vi "Begin.vi"(8 "error in":errorcluster) -> (0 "error out":errorcluster)   [LabVIEW 2015]
doc: "Called before other user functions, this VI is expected to open initial I/O refnums, load in file data, and do all program initialization. Notice that the <B>error out</B> terminal is simply used for data flow. Wiring it to other structures or subVIs ensures that this VI runs first."
uses:
  <vilib>/Rock Robotics/WPI/DriverStation/WPI_DriverStationRobotMode2.ctl
  <vilib>/Rock Robotics/WPI/Joystick/WPI_JoystickDeviceEnum.ctl
  <vilib>/Rock Robotics/WPI/Solenoid/WPI_SolenoidChannel.ctl
  <vilib>/Rock Robotics/SystemInterfaces/AI/FPGA_AIChannel.ctl
  <vilib>/Rock Robotics/SystemInterfaces/DIO/FPGA_DIOChannel.ctl
  <vilib>/Rock Robotics/WPI/CAN/TalonSRX/WPI_CANTalonSRX_APIControlMode.ctl
  <vilib>/Rock Robotics/WPI/CAN/TalonSRX/WPI_CANTalonSRX_BrakeOverride.ctl
  <vilib>/Rock Robotics/SystemInterfaces/i2clib/i2c_bus.ctl
  <vilib>/Rock Robotics/WPI/AnalogOutput/WPI_AnalogOutputChannel.ctl
  navX-MXP Library/COMMON/TypeDefs/Value TypeDefs/navX Update Rate.ctl
  navX-MXP Library/COMMON/TypeDefs/Value TypeDefs/navX Interface Protocol.ctl
  <vilib>/Rock Robotics/SystemInterfaces/spilib/spi_bus.ctl
  Robot Global Data.vi
  <vilib>/Rock Robotics/WPI/Solenoid/WPI_SolenoidOpenSingle.vi
  <vilib>/Rock Robotics/WPI/Counter/WPI_CounterDigitalInputToDigitalSource.vi
  <vilib>/Rock Robotics/WPI/MotorControl/WPI_MotorControlOpenCANTalonSRX.vi
  <vilib>/Rock Robotics/WPI/Ultrasonic/WPI_SonarSRF04DigitalOpen.vi
  <vilib>/Rock Robotics/WPI/Ultrasonic/WPI_SonarSRF04DigitalRefNum Registry Set.vi
  <vilib>/Rock Robotics/WPI/Utilities/WPI_GetSetVariantRefNum.vi
  <vilib>/Rock Robotics/WPI/Camera/WPI_CameraWhite Balance Values.ctl
  <vilib>/Rock Robotics/WPI/Camera/WPI_CameraExposure Values.ctl
  <vilib>/Rock Robotics/WPI/Accelerometer/ADXL345 Range.ctl
  <vilib>/Rock Robotics/WPI/Accelerometer/WPI_AccelerometerADXL345 Axes.ctl
  <vilib>/Rock Robotics/WPI/RobotDrive/WPI_RobotDriveOpen2MotorWithExistingMotors.vi
  navX-MXP Library/navX-MXP IMU.lvlib
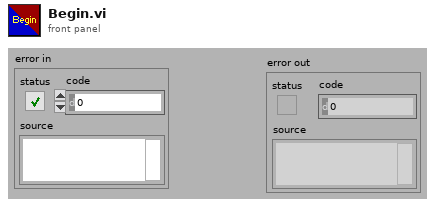
[diagram p1: front panel]
types:
  T1 = typedef "FPGA_AIChannel.ctl" = enum8{"AI 0", "AI 1", "AI 2", "AI 3", "AI MXP 0", "AI MXP 1", "AI MXP 2", "AI MXP 3", "Invalid"}
  T2 = typedef "FPGA_DIOChannel.ctl" = enum8{"DIO 0", "DIO 1", "DIO 2", "DIO 3", "DIO 4", "DIO 5", "DIO 6", "DIO 7", "DIO 8", "DIO 9", "DIO MXP 0", "DIO MXP 1", "DIO MXP 2", "DIO MXP 3", "DIO MXP 4", "DIO MXP 5", "DIO MXP 6", "DIO MXP 7", "DIO MXP 8", "DIO MXP 9", "DIO MXP 10", "DIO MXP 11", "DIO MXP 12", "DIO MXP 13", "DIO MXP 14", "DIO MXP 15", "Invalid"}
  T3 = typedef "WPI_AnalogOutputChannel.ctl" = enum8{"AO MXP 0", "AO MXP 1", "Invalid"}
  T4 = typedef "i2c_bus.ctl" = enum16{"I2C On-Board", "I2C MXP", "Invalid"}
  T5 = typedef "WPI_SolenoidChannel.ctl" = enum8{"Solenoid 0", "Solenoid 1", "Solenoid 2", "Solenoid 3", "Solenoid 4", "Solenoid 5", "Solenoid 6", "Solenoid 7", "Invalid"}
  T6 = typedef "WPI_CANTalonSRX_BrakeOverride.ctl" = enum8{"No Override", "Override to Coast", "Override to Brake"}
  T7 = typedef "WPI_CANTalonSRX_APIControlMode.ctl" = enum8{"Percent VBus", "Speed", "Position", "Slave", "Unchanged / Invalid", "Voltage Compensation", "Current", "Motion Profile"}
  T8 = typedef "WPI_JoystickDeviceEnum.ctl" = enum16{"USB 0", "USB 1", "USB 2", "USB 3", "USB 4", "USB 5"}
  T9 = typedef "WPI_DriverStationRobotMode2.ctl" = enum16{"Autonomous Disabled", "Autonomous Enabled", "Teleop Disabled", "Teleop Enabled", "Disconnected", "Finish", "Test Disabled", "Test Enabled", "Emergency Stopped"}
  T10 = typedef "WPI_CameraExposure Values.ctl" = enum16{"Auto", "Flicker-free 50 Hz", "Flicker-free 60 Hz", "Hold current", "Custom"}
  T11 = typedef "WPI_CameraWhite Balance Values.ctl" = enum16{"Auto", "Fixed indoor", "Fixed outdoor 1", "Fixed outdoor 2", "Fixed fluorescent 1", "Fixed fluorescent 2", "Hold current", "Custom"}
  T12 = typedef "WPI_CameraDevRef.ctl" = cluster{"Camera Address":string, "CameraStatus":errorcluster}
  T13 = typedef "WPI_SolenoidDevRef.ctl" = cluster{"DevStatus":errorcluster, "Pneumatics Control Module":u8, "Forward Solenoid Channel":T5, "Reverse Solenoid Channel":T5}
  T14 = typedef "WPI_MotorControlDeviceRef.ctl" = cluster{"DeviceStatus":errorcluster, "Type":T15, "PWM":cluster{"PWM Channel":T16, "DeadBand":T17}, "CAN":cluster{"Device Number":u8, "Control Mode":T18, "Semaphore":T19, "Max Vout":dbl, "TalonSRX Control Mode":T7}, "Invert":bool}
  T15 = typedef "WPI_MotorControlType.ctl" = enum16{"PWM", "CAN", "CANTalonSRX"}
  T16 = typedef "FPGA_DIOPWMChannel.ctl" = enum8{"PWM 0", "PWM 1", "PWM 2", "PWM 3", "PWM 4", "PWM 5", "PWM 6", "PWM 7", "PWM 8", "PWM 9", "PWM MXP 0", "PWM MXP 1", "PWM MXP 2", "PWM MXP 3", "PWM MXP 4", "PWM MXP 5", "PWM MXP 6", "PWM MXP 7", "PWM MXP 8", "PWM MXP 9", "Invalid"}
  T17 = typedef "WPI_PWMDeadband.ctl" = cluster{"Name":string, "maxPositivePwm":i32, "minPositivePwm":i32, "centerPwm":i32, "maxNegativePwm":i32, "minNegativePwm":i32, "angularRange":u16}
  T18 = typedef "WPI_CANJaguar_ControlMode.ctl" = enum8{"Percent VBus", "Current", "Speed", "Position", "Voltage"}
  T19 = typedef "Semaphore RefNum" = refnum<k1>
  T20 = typedef "WPI_DigitalInputDevRef.ctl" = cluster{"DevStatus":errorcluster, "DIO Channel":T2}
  T21 = typedef "WPI_CompressorDevRef.ctl" = cluster{"DevStatus":errorcluster, "Pneumatics Control Module":u8}
  T22 = typedef "FPGA_CounterEncoderSourceConvertionLVSourceType.ctl" = cluster{"DevStatus":errorcluster, "AnalogTriggerMode?":bool, "DigitalMode":cluster{"DIO Channel":T23}, "AnalogTriggerMode":cluster{"AnalogTriggerIndex":T24, "OutputType":T25}}
  T23 = typedef "FPGA_DIODigitalSourceChannel.ctl" = enum8{"DIO 0", "DIO 1", "DIO 2", "DIO 3", "DIO 4", "DIO 5", "DIO 6", "DIO 7", "DIO 8", "DIO 9", "DIO MXP 0", "DIO MXP 1", "DIO MXP 2", "DIO MXP 3", "DIO MXP 4", "DIO MXP 5", "DIO MXP 6", "DIO MXP 7", "DIO MXP 8", "DIO MXP 9", "DIO MXP 10", "DIO MXP 11", "DIO MXP 12", "DIO MXP 13", "DIO MXP 14", "DIO MXP 15", "Disabled"}
  T24 = typedef "FPGA_AnalogTriggerIndex.ctl" = enum8{"Trig 0", "Trig 1", "Trig 2", "Trig 3", "Trig 4", "Trig 5", "Trig 6", "Trig 7", "Invalid"}
  T25 = typedef "FPGA_AnalogTriggerOutType.ctl" = enum16{"InWindow", "TriggerState", "Rising", "Falling"}
  T26 = typedef "WPI_EncoderDevRef.ctl" = cluster{"DevStatus":errorcluster, "EncoderIndex":T27, "CounterIndex":T28, "DistancePerCount":dbl, "Decoding Type":T29}
  T27 = typedef "FPGA_EncoderIdx.ctl" = enum8{"Enc 0", "Enc 1", "Enc 2", "Enc 3", "Enc 4", "Enc 5", "Enc 6", "Enc 7", "Invalid"}
  T28 = typedef "FPGA_CounterCtrSystemIndex.ctl" = enum8{"Ctr 0", "Ctr 1", "Ctr 2", "Ctr 3", "Ctr 4", "Ctr 5", "Ctr 6", "Ctr 7", "Invalid"}
  T29 = typedef "WPI_EncoderType.ctl" = enum16{"1x", "2x", "4x"}
  T30 = typedef "WPI_AccelerometerADXL345 Axes.ctl" = cluster{"X-Axis":bool, "Y-Axis":bool, "Z-Axis":bool}
  T31 = typedef "spi_bus.ctl" = enum16{"SPI On-Board, CS0", "SPI On-Board, CS1", "SPI On-Board, CS2", "SPI On-Board, CS3", "SPI MXP", "Invalid"}
  T32 = typedef "navX-MXP IMU.lvlib/navX Interface Protocol.ctl" = enum16{"SPI", "I2C"}
  T33 = typedef "navX-MXP IMU.lvlib/navX Update Rate.ctl" = u8
  T34 = typedef "WPI_I2CDevRef.ctl" = cluster{"DevStatus":errorcluster, "Device Address":u8, "Handle":i32, "I2C Bus":T4}
  T35 = typedef "ADXL345 Range.ctl" = u8
  T36 = typedef "WPI_AccelerometerDevRef.ctl" = cluster{"DevStatus":errorcluster, "Scaling":T37, "Analog Channels":T38, "I2C Bus":T4, "SPI Bus":T31, "Accel Range":T35, "ADXL Axes":T30, "Handle":i32, "Device Address":u8, "Accel Type":enum16{"Analog", "ADXL345 I2C", "ADXL345 SPI", "Internal", "ADXL362 SPI"}}
  T37 = typedef "WPI_AccelerometerScaling.ctl" = cluster{"Gain (VoltsPerG)":dbl, "Center Voltage":dbl}
  T38 = typedef "WPI_AccelerometerAnalogChannels.ctl" = cluster{"X-Axis":T1, "Y-Axis":T1, "Z-Axis":T1}
  T39 = typedef "navX-MXP IMU.lvlib/navX Device TypeDef.ctl" = cluster{"navX Interface Protocol":T32, "navX Interface Protocol TypeDefs":cluster{"SPIDevRef":T40, "I2CDevRef":T34}, "navX System Information":cluster{"Board Information":T41, "Status":T42, "Offsets":T46}, "navX Common Information":cluster{"Update Rate (4Hz-60Hz)":T33, "refnum name":string, "error":errorcluster}}
  T40 = typedef "WPI_SPIDevRef.ctl" = cluster{"DevStatus":errorcluster, "Handle":i32, "SPI Bus":T31}
  T41 = typedef "navX-MXP IMU.lvlib/navX Board Information.ctl" = cluster{"WhoAmI (50 | 0x32)":u8, "Board Revision":u8, "Firmware Major Version":u8, "Firmware Minor Version":u8}
  T42 = typedef "navX-MXP IMU.lvlib/navX Status Data.ctl" = cluster{"Update Rate Hz":u8, "Accelerometer Full-Scale Range":u8, "Gyro Full-Scale Range":u16, "NAVX_OP_STATUS":T43, "NAVX_CAL_STATUS":T44, "NAVX_SELFTEST_STATUS":u8, "NAVX_SENSOR_STATUS":T45}
  T43 = typedef "navX-MXP IMU.lvlib/navX NAVX_OP_STATUS.ctl" = u8
  T44 = typedef "navX-MXP IMU.lvlib/navX NAVX_CAL_STATUS.ctl" = u8
  T45 = typedef "navX-MXP IMU.lvlib/navX NAVX_SENSOR_STATUS.ctl" = cluster{"MOVING":bool, "YAW_STABLE":bool, "MAG_DISTURBANCE":bool, "ALTITUDE_VALID":bool, "SEALEVEL_PRESS_SET":bool, "FUSED_HEADING_VALID":bool}
  T46 = typedef "navX-MXP IMU.lvlib/navX Offsets Data.ctl" = cluster{"Yaw":dbl, "Quat W":dbl, "Quat X":dbl, "Quat Y":dbl, "Quat Z":dbl}
  T47 = typedef "WPI_AnalogChannelDevRef.ctl" = cluster{"DevStatus":errorcluster, "Analog Channel":T1}
  T48 = typedef "WPI_PotentiometerDevRef.ctl" = cluster{"DevStatus":errorcluster, "Analog Channel":T1, "Invert Output":bool}
  T49 = typedef "WPI_JoystickDevRef.ctl" = cluster{"Device":T8}
  T50 = typedef "WPI_RobotDriveDevRef.ctl" = cluster{"DevStatus":errorcluster, "Motors[]":T14[], "Square Inputs":bool, "Max Output":dbl}
  T51 = typedef "WPI_UltrasonicDeviceRef.ctl" = cluster{"DevStatus":errorcluster, "Ping Channel":T2, "Echo Channel":T2, "CntIndex":T28}
  T52 = typedef "WPI_AOChannelDevRef.ctl" = cluster{"DevStatus":errorcluster, "AO Channel":T3}
  T53 = typedef "WPI_DigitalOutputDevRef.ctl" = cluster{"DIO Channel":T2, "DevStatus":errorcluster}
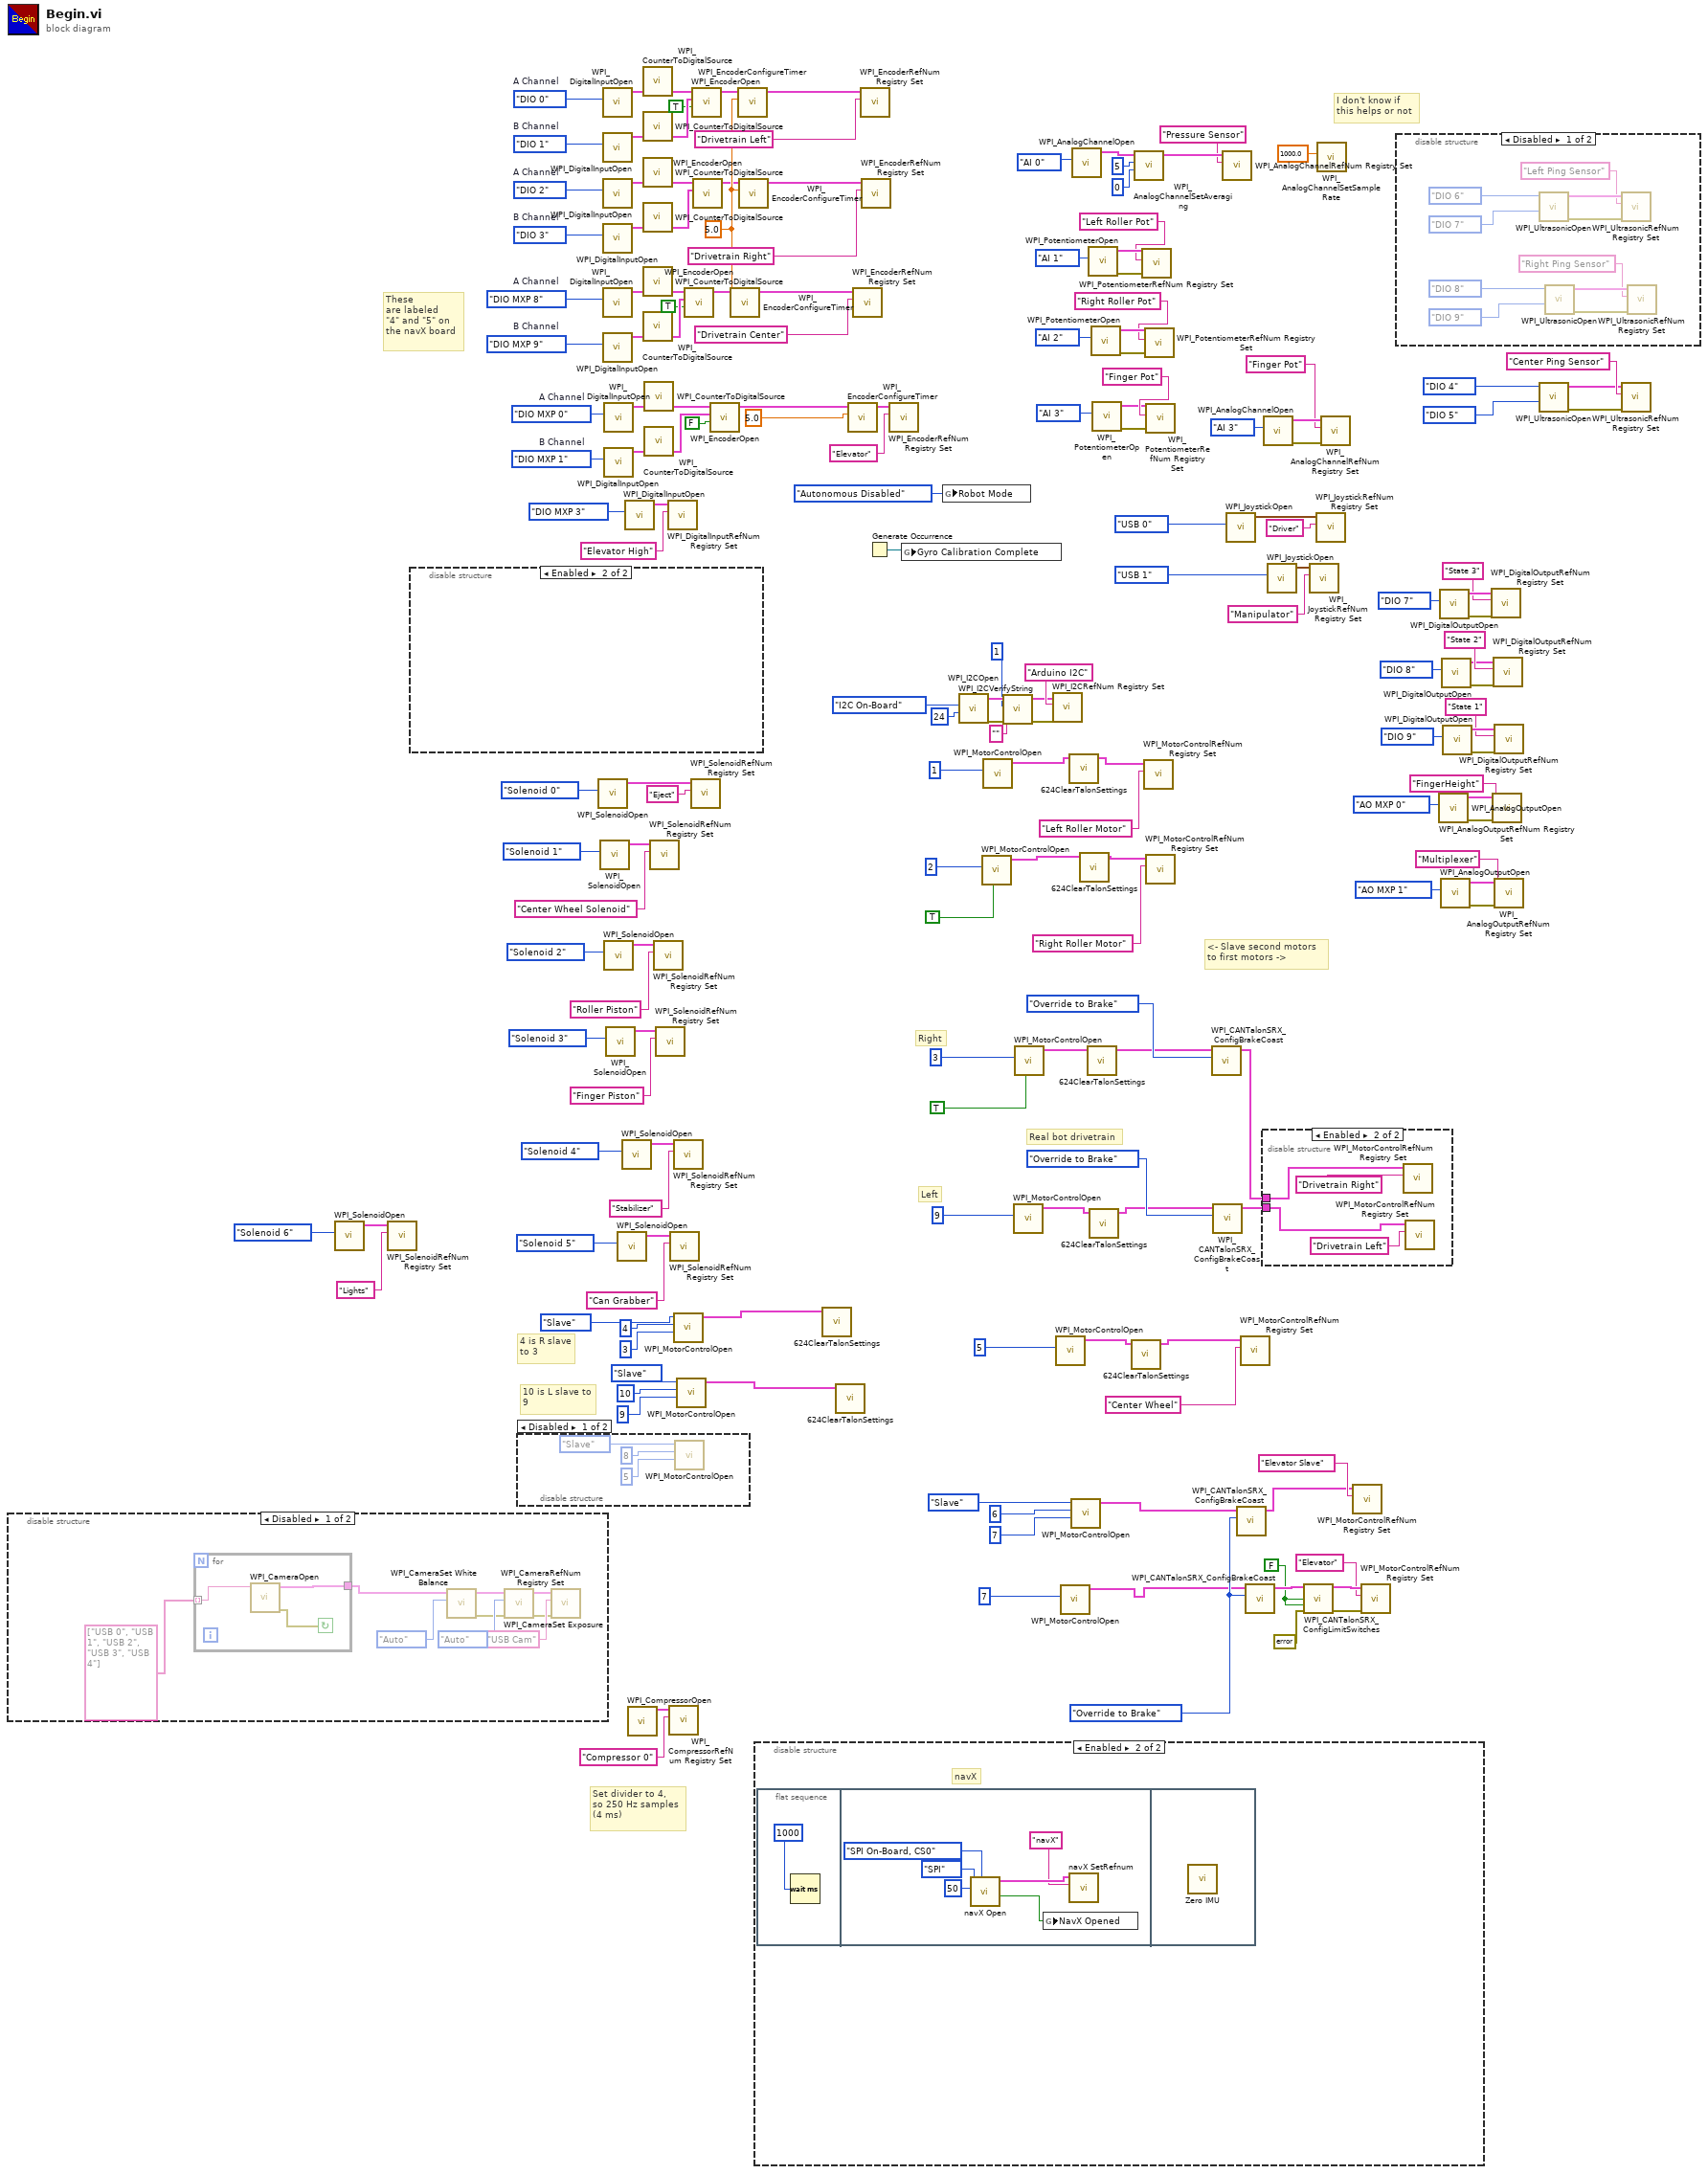
[diagram p0: block diagram]
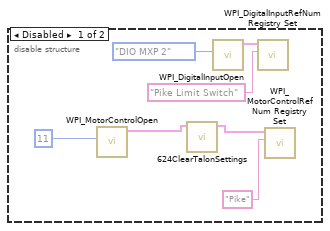
[diagram p2: hidden frame]
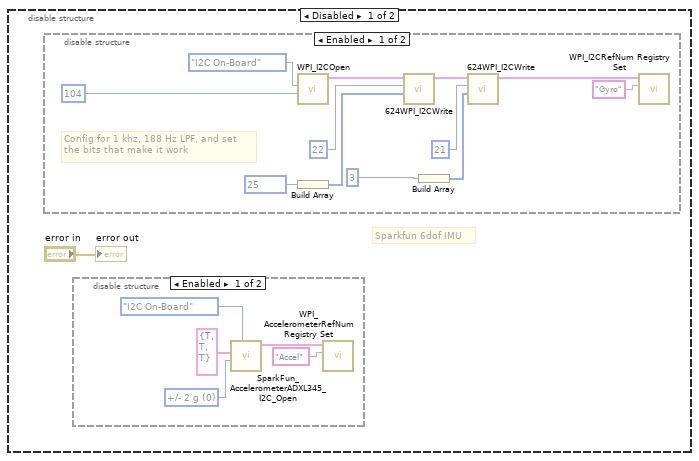
[diagram p5: hidden frame]
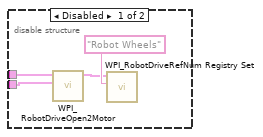
[diagram p9: hidden frame]
diagram:
  w41 = FPGA_DIOChannel."DIO MXP 9"  # B Channel
  w42 = FPGA_DIOChannel."DIO MXP 8"  # A Channel
  w66 = FALSE ("Forward Limit Switch Normally Open")
  w64 = WPI_CANTalonSRX_BrakeOverride."Override to Brake" ("Brake / Coast Mode")
  w94 = FPGA_DIOChannel."DIO MXP 1"  # B Channel
  w95 = FPGA_DIOChannel."DIO MXP 0"  # A Channel
  w122 = FPGA_DIOChannel."DIO 3"  # B Channel
  w125 = FPGA_DIOChannel."DIO 2"  # A Channel
  w131 = FPGA_DIOChannel."DIO 0"  # A Channel
  w134 = FPGA_DIOChannel."DIO 1"  # B Channel
  w139 = 5.0 ("Minimum Rate")
  # "10 is L slave to\n9"
  # "4 is R slave\nto 3"
  # "These \nare labeled\n\"4\" and \"5\" on \nthe navX board"
  # "<- Slave second motors\nto first motors ->"
  # "Left"
  # "Right"
  # "Real bot drivetrain"
  # "I don't know if \nthis helps or not"
  # "Set divider to 4, \nso 250 Hz samples\n(4 ms)"
  n1 = disable-structure shown="Disabled" {
    frame Disabled {
      n2 = for {
        tunnel: string[] ["USB 0", "USB 1", "USB 2", "USB 3", "USB 4"] -> [w191] mode=indexing
        tunnel: [w190] -> w180
        stop <- w189 continue-if-true
        n3 = call <vilib>:"WPI_CameraOpen.vi"("Camera Address"=w191) -> ("error out"=w189:errorcluster, "CameraDevRef"=w190:T12)  [unwired: 9 in]
      }
      n4 = call <vilib>:"WPI_CameraSet White Balance.vi"("White Balance"=WPI_CameraWhite_Balance_Values."Auto", "CameraDevRef"=w180) -> ("error out"=w183:errorcluster, "CameraDevRef Out"=w187:T12)  [unwired: 8 in]
      n5 = call <vilib>:"WPI_CameraSet Exposure.vi"("error in (no error)"=w183, "Exposure"=WPI_CameraExposure_Values."Auto", "CameraDevRef"=w187) -> ("error out"=w182:errorcluster, "CameraDevRef Out"=w185:T12)  [unwired: 7 in]
      n6 = call <vilib>:"WPI_CameraRefNum Registry Set.vi"("error in (no error)"=w182, "refnum name"="USB Cam", "CameraDevRef"=w185) -> ()  [unwired: 7 in, 2 out]
    }
    frame Enabled {
    }
  }
  n7 = call-poly <vilib>:"WPI_SolenoidOpen.vi"("Solenoid Channel"=WPI_SolenoidChannel."Solenoid 6") -> ("SolenoidDevRef"=w39:T13)  [unwired: 9 in, 1 out]
  n8 = call <vilib>:"WPI_SolenoidRefNum Registry Set.vi"("refnum name"="Lights", "SolenoidDevRef"=w39) -> ()  [unwired: 8 in, 2 out]
  n9 = disable-structure shown="Enabled" {
    frame Disabled {
      n10 = call-poly <vilib>:"WPI_MotorControlOpen.vi"("Device Number"=u8 11) -> ("MotorControlDeviceRef"=w194:T14)  [unwired: 9 in, 1 out]
      n11 = call "624ClearTalonSettings.vi"("CAN Talon SRX Ref Out"=w194) -> ("CAN Talon SRX Ref Out 2"=w193:T14)  [unwired: 10 in]
      n12 = call <vilib>:"WPI_DigitalInputOpen.vi"("DIO Channel"=FPGA_DIOChannel."DIO MXP 2") -> ("DigitalInputDevRef"=w196:T20)  [unwired: 9 in, 1 out]
      n13 = call <vilib>:"WPI_DigitalInputRefNum Registry Set.vi"("refnum name"="Pike Limit Switch", "DigitalInputDevRef"=w196) -> ()  [unwired: 8 in, 2 out]
      n14 = call <vilib>:"WPI_MotorControlRefNum Registry Set.vi"("refnum name"="Pike", "MotorControlDevRef"=w193) -> ()  [unwired: 8 in, 2 out]
    }
    frame Enabled {
    }
  }
  n15 = disable-structure shown="Disabled" {
    frame Disabled {
      n16 = call-poly <vilib>:"WPI_MotorControlOpen.vi"("Master Device Number"=u8 5, "Device Number"=u8 8, "Control Mode"=WPI_CANTalonSRX_APIControlMode."Slave") -> ()  [unwired: 7 in, 2 out]
    }
    frame Enabled {
    }
  }
  n17 = call-poly <vilib>:"WPI_SolenoidOpen.vi"("Solenoid Channel"=WPI_SolenoidChannel."Solenoid 0") -> ("SolenoidDevRef"=w108:T13)  [unwired: 9 in, 1 out]
  n18 = call-poly <vilib>:"WPI_SolenoidOpen.vi"("Solenoid Channel"=WPI_SolenoidChannel."Solenoid 1") -> ("SolenoidDevRef"=w107:T13)  [unwired: 9 in, 1 out]
  n19 = call <vilib>:"WPI_DigitalInputOpen.vi"("DIO Channel"=w131) -> ("DigitalInputDevRef"=w132:T20)  [unwired: 1 in, 9 out]
  n20 = call <vilib>:"WPI_DigitalInputOpen.vi"("DIO Channel"=w134) -> ("DigitalInputDevRef"=w135:T20)  [unwired: 1 in, 9 out]
  n21 = call <vilib>:"WPI_DigitalInputOpen.vi"("DIO Channel"=w125) -> ("DigitalInputDevRef"=w126:T20)  [unwired: 1 in, 9 out]
  n22 = call <vilib>:"WPI_DigitalInputOpen.vi"("DIO Channel"=w122) -> ("DigitalInputDevRef"=w123:T20)  [unwired: 1 in, 9 out]
  n23 = call <vilib>:"WPI_DigitalInputOpen.vi"("DIO Channel"=w42) -> ("DigitalInputDevRef"=w140:T20)  [unwired: 1 in, 9 out]
  n24 = call <vilib>:"WPI_DigitalInputOpen.vi"("DIO Channel"=w41) -> ("DigitalInputDevRef"=w142:T20)  [unwired: 1 in, 9 out]
  n25 = call <vilib>:"WPI_DigitalInputOpen.vi"("DIO Channel"=w95) -> ("DigitalInputDevRef"=w156:T20)  [unwired: 1 in, 9 out]
  n26 = call <vilib>:"WPI_DigitalInputOpen.vi"("DIO Channel"=w94) -> ("DigitalInputDevRef"=w158:T20)  [unwired: 1 in, 9 out]
  n27 = call-poly <vilib>:"WPI_SolenoidOpen.vi"("Solenoid Channel"=WPI_SolenoidChannel."Solenoid 2") -> ("SolenoidDevRef"=w109:T13)  [unwired: 9 in, 1 out]
  n28 = call-poly <vilib>:"WPI_SolenoidOpen.vi"("Solenoid Channel"=WPI_SolenoidChannel."Solenoid 3") -> ("SolenoidDevRef"=w111:T13)  [unwired: 9 in, 1 out]
  n29 = call-poly <vilib>:"WPI_SolenoidOpen.vi"("Solenoid Channel"=WPI_SolenoidChannel."Solenoid 5") -> ("SolenoidDevRef"=w45:T13)  [unwired: 9 in, 1 out]
  n30 = call-poly <vilib>:"WPI_SolenoidOpen.vi"("Solenoid Channel"=WPI_SolenoidChannel."Solenoid 4") -> ("SolenoidDevRef"=w114:T13)  [unwired: 9 in, 1 out]
  n31 = call <vilib>:"WPI_DigitalInputOpen.vi"("DIO Channel"=FPGA_DIOChannel."DIO MXP 3") -> ("DigitalInputDevRef"=w164:T20)  [unwired: 9 in, 1 out]
  n32 = call <vilib>:"WPI_CompressorOpen.vi"() -> ("CompressorDevRef"=w173:T21)  [unwired: 14 in, 1 out]
  n33 = call-poly <vilib>:"WPI_CounterToDigitalSource.vi"("DigitalInputDevRef"=w132) -> ("Digital Source"=w133:T22)  [unwired: 6 out]
  n34 = call-poly <vilib>:"WPI_CounterToDigitalSource.vi"("DigitalInputDevRef"=w135) -> ("Digital Source"=w136:T22)  [unwired: 6 out]
  n35 = call-poly <vilib>:"WPI_CounterToDigitalSource.vi"("DigitalInputDevRef"=w126) -> ("Digital Source"=w127:T22)  [unwired: 6 out]
  n36 = call-poly <vilib>:"WPI_CounterToDigitalSource.vi"("DigitalInputDevRef"=w123) -> ("Digital Source"=w124:T22)  [unwired: 6 out]
  n37 = call-poly <vilib>:"WPI_CounterToDigitalSource.vi"("DigitalInputDevRef"=w140) -> ("Digital Source"=w141:T22)  [unwired: 6 out]
  n38 = call-poly <vilib>:"WPI_CounterToDigitalSource.vi"("DigitalInputDevRef"=w142) -> ("Digital Source"=w143:T22)  [unwired: 6 out]
  n39 = call-poly <vilib>:"WPI_CounterToDigitalSource.vi"("DigitalInputDevRef"=w156) -> ("Digital Source"=w157:T22)  [unwired: 6 out]
  n40 = call-poly <vilib>:"WPI_CounterToDigitalSource.vi"("DigitalInputDevRef"=w158) -> ("Digital Source"=w159:T22)  [unwired: 6 out]
  n41 = call <vilib>:"WPI_SolenoidRefNum Registry Set.vi"("refnum name"="Center Wheel Solenoid", "SolenoidDevRef"=w107) -> ()  [unwired: 8 in, 2 out]
  n42 = call <vilib>:"WPI_SolenoidRefNum Registry Set.vi"("refnum name"="Roller Piston", "SolenoidDevRef"=w109) -> ()  [unwired: 8 in, 2 out]
  n43 = call <vilib>:"WPI_SolenoidRefNum Registry Set.vi"("refnum name"="Finger Piston", "SolenoidDevRef"=w111) -> ()  [unwired: 8 in, 2 out]
  n44 = call <vilib>:"WPI_DigitalInputRefNum Registry Set.vi"("refnum name"="Elevator High", "DigitalInputDevRef"=w164) -> ()  [unwired: 8 in, 2 out]
  n45 = call <vilib>:"WPI_CompressorRefNum Registry Set.vi"("refnum name"="Compressor 0", "CompressorDevRef"=w173) -> ()  [unwired: 8 in, 2 out]
  n46 = call <vilib>:"WPI_SolenoidRefNum Registry Set.vi"("refnum name"="Can Grabber", "SolenoidDevRef"=w45) -> ()  [unwired: 8 in, 2 out]
  n47 = call <vilib>:"WPI_SolenoidRefNum Registry Set.vi"("refnum name"="Stabilizer", "SolenoidDevRef"=w114) -> ()  [unwired: 8 in, 2 out]
  n48 = call-poly <vilib>:"WPI_MotorControlOpen.vi"("Master Device Number"=u8 3, "Device Number"=u8 4, "Control Mode"=WPI_CANTalonSRX_APIControlMode."Slave") -> ("MotorControlDeviceRef"=w53:T14)  [unwired: 7 in, 1 out]
  n49 = call-poly <vilib>:"WPI_MotorControlOpen.vi"("Master Device Number"=u8 9, "Device Number"=u8 10, "Control Mode"=WPI_CANTalonSRX_APIControlMode."Slave") -> ("MotorControlDeviceRef"=w52:T14)  [unwired: 7 in, 1 out]
  n50 = call <vilib>:"WPI_EncoderOpen.vi"("Invert Direction (False)"=TRUE, "BSource"=w143, "ASource"=w141) -> ("EncoderDevRef"=w144:T26)  [unwired: 5 in, 3 out]
  n51 = call <vilib>:"WPI_SolenoidRefNum Registry Set.vi"("refnum name"="Eject", "SolenoidDevRef"=w108) -> ()  [unwired: 8 in, 2 out]
  n52 = call <vilib>:"WPI_EncoderOpen.vi"("Invert Direction (False)"=TRUE, "BSource"=w136, "ASource"=w133) -> ("EncoderDevRef"=w137:T26)  [unwired: 5 in, 3 out]
  n53 = call <vilib>:"WPI_EncoderOpen.vi"("BSource"=w124, "ASource"=w127) -> ("EncoderDevRef"=w128:T26)  [unwired: 6 in, 3 out]
  n54 = call <vilib>:"WPI_EncoderOpen.vi"("Invert Direction (False)"=FALSE, "BSource"=w159, "ASource"=w157) -> ("EncoderDevRef"=w160:T26)  [unwired: 5 in, 3 out]
  n55 = call <vilib>:"WPI_EncoderConfigureTimer.vi"("Minimum Rate"=w139, "EncoderDevRef"=w144) -> ("EncoderDevRef"=w145:T26)  [unwired: 8 in, 1 out]
  n56 = call <vilib>:"WPI_EncoderConfigureTimer.vi"("Minimum Rate"=w139, "EncoderDevRef"=w137) -> ("EncoderDevRef"=w138:T26)  [unwired: 8 in, 1 out]
  n57 = call <vilib>:"WPI_EncoderConfigureTimer.vi"("Minimum Rate"=w139, "EncoderDevRef"=w128) -> ("EncoderDevRef"=w129:T26)  [unwired: 8 in, 1 out]
  n58 = disable-structure shown="Enabled" {
    frame Disabled {
      # "Sparkfun 6dof IMU"
      n59 = disable-structure shown="Enabled" {
        frame Enabled {
          # "Config for 1 khz, 188 Hz LPF, and set\nthe bits that make it work"
          n60 = call <vilib>:"WPI_I2COpen.vi"("Device Address"=104, "I2C Bus"=i2c_bus."I2C On-Board") -> ("I2CDevRef"=w218:T34)  [unwired: 8 in, 1 out]
          n61 = Build Array(u8 25) -> (w215:u8[])
          n62 = call "624WPI_I2CWrite.vi"("I2CDataToSend"=w215, "I2CRegister"=u8 22, "I2CDevRef"=w218) -> ("I2CDevRef"=w219:T34)  [unwired: 7 in, 1 out]
          n63 = Build Array(u8 3) -> (w212:u8[])
          n64 = call "624WPI_I2CWrite.vi"("I2CDataToSend"=w212, "I2CRegister"=u8 21, "I2CDevRef"=w219) -> ("I2CDevRef"=w208:T34)  [unwired: 7 in, 1 out]
          n65 = call <vilib>:"WPI_I2CRefNum Registry Set.vi"("refnum name"="Gyro", "I2CDevRef"=w208) -> ()  [unwired: 8 in, 2 out]
        }
        frame Disabled {
        }
      }
      n66 = disable-structure shown="Enabled" {
        frame Enabled {
          w206 = T35 0 items=["+/- 2 g", "+/- 4 g", "+/- 8 g", "+/- 16 g"] ("Accel Range")
          n67 = call "SparkFun_AccelerometerADXL345_I2C_Open.vi"("I2C Bus"=i2c_bus."I2C On-Board", "Accel Range"=w206, "ADXL345 Axes"=T30 {"X-Axis"=TRUE, "Y-Axis"=TRUE, "Z-Axis"=TRUE}) -> ("AccelerometerDevRef"=w207:T36)  [unwired: 7 in, 1 out]
          n68 = call <vilib>:"WPI_AccelerometerRefNum Registry Set.vi"("refnum name"="Accel", "AccelerometerDevRef"=w207) -> ()  [unwired: 8 in, 2 out]
        }
        frame Disabled {
        }
      }
      "error out" <- "error in"
    }
    frame Enabled {
      # "navX"
      n69 = flat-sequence {
        frame #0 {
          n70 = Wait (ms)(milliseconds to wait=u32 1000) -> ()  [unwired: 1 out]
        }
        frame #1 {
          n71 = call "navX Open.vi"("SPI Bus"=spi_bus."SPI On-Board, CS0", "Update Rate (4Hz-60Hz)"=T33 50, "navX Interface Protocol"=navX_Interface_Protocol."SPI") -> ("Opened?"=w224:bool, "navX Device TypeDef"=w226:T39)  [unwired: 6 in, 1 out]
          n72 = global write "Robot Global Data.vi" "NavX Opened"(w224) -> ()
          n73 = call "navX SetRefnum.vi"("refnum name"="navX", "navX Device TypeDef"=w226) -> ()  [unwired: 8 in, 2 out]
        }
        frame #2 {
          n74 = call "Zero IMU.vi"() -> ()  [unwired: 12 in]
        }
      }
    }
  }
  n75 = call "624ClearTalonSettings.vi"("CAN Talon SRX Ref Out"=w53) -> ()  [unwired: 10 in, 1 out]
  n76 = call "624ClearTalonSettings.vi"("CAN Talon SRX Ref Out"=w52) -> ()  [unwired: 10 in, 1 out]
  n77 = call <vilib>:"WPI_EncoderConfigureTimer.vi"("Minimum Rate"=5.0, "EncoderDevRef"=w160) -> ("EncoderDevRef"=w161:T26)  [unwired: 8 in, 1 out]
  n78 = call <vilib>:"WPI_EncoderRefNum Registry Set.vi"("refnum name"="Drivetrain Center", "EncoderDevRef"=w145) -> ()  [unwired: 8 in, 2 out]
  n79 = call <vilib>:"WPI_EncoderRefNum Registry Set.vi"("refnum name"="Drivetrain Left", "EncoderDevRef"=w138) -> ()  [unwired: 8 in, 2 out]
  n80 = call <vilib>:"WPI_EncoderRefNum Registry Set.vi"("refnum name"="Drivetrain Right", "EncoderDevRef"=w129) -> ()  [unwired: 8 in, 2 out]
  n81 = Generate Occurrence() -> (w48:refnum<k4>)
  n82 = call <vilib>:"WPI_EncoderRefNum Registry Set.vi"("refnum name"="Elevator", "EncoderDevRef"=w161) -> ()  [unwired: 8 in, 2 out]
  n83 = global write "Robot Global Data.vi" "Gyro Calibration Complete"(w48) -> ()
  n84 = global write "Robot Global Data.vi" "Robot Mode"(WPI_DriverStationRobotMode2."Autonomous Disabled" ("Robot Mode")) -> ()
  n85 = call <vilib>:"WPI_I2COpen.vi"("Device Address"=u8 24, "I2C Bus"=i2c_bus."I2C On-Board") -> ("error out"=w31:errorcluster, "I2CDevRef"=w34:T34)  [unwired: 8 in]
  n86 = call-poly <vilib>:"WPI_MotorControlOpen.vi"("Invert"=TRUE, "Device Number"=u8 2) -> ("MotorControlDeviceRef"=w56:T14)  [unwired: 8 in, 1 out]
  n87 = call-poly <vilib>:"WPI_MotorControlOpen.vi"("Device Number"=u8 1) -> ("MotorControlDeviceRef"=w54:T14)  [unwired: 9 in, 1 out]
  n88 = call <vilib>:"WPI_I2CVerifyString.vi"("error in (no error)"=w31, "Expected"="", "Register Address"=u8 1, "I2CDevRef"=w34) -> ("error out"=w32:errorcluster, "I2CDevRef"=w33:T34)  [unwired: 6 in]
  n89 = call-poly <vilib>:"WPI_MotorControlOpen.vi"("Device Number"=u8 9) -> ("MotorControlDeviceRef"=w60:T14)  [unwired: 9 in, 1 out]
  n90 = call-poly <vilib>:"WPI_MotorControlOpen.vi"("Invert"=TRUE, "Device Number"=u8 3) -> ("MotorControlDeviceRef"=w58:T14)  [unwired: 8 in, 1 out]
  n91 = call <vilib>:"WPI_I2CRefNum Registry Set.vi"("error in (no error)"=w32, "refnum name"="Arduino I2C", "I2CDevRef"=w33) -> ()  [unwired: 7 in, 2 out]
  n92 = call-poly <vilib>:"WPI_MotorControlOpen.vi"("Device Number"=u8 5) -> ("MotorControlDeviceRef"=w62:T14)  [unwired: 9 in, 1 out]
  n93 = call-poly <vilib>:"WPI_MotorControlOpen.vi"("Device Number"=u8 7) -> ("MotorControlDeviceRef"=w49:T14)  [unwired: 9 in, 1 out]
  n94 = call "624ClearTalonSettings.vi"("CAN Talon SRX Ref Out"=w54) -> ("CAN Talon SRX Ref Out 2"=w55:T14)  [unwired: 10 in]
  n95 = call-poly <vilib>:"WPI_MotorControlOpen.vi"("Master Device Number"=u8 7, "Device Number"=u8 6, "Control Mode"=WPI_CANTalonSRX_APIControlMode."Slave") -> ("MotorControlDeviceRef"=w50:T14)  [unwired: 7 in, 1 out]
  n96 = call <vilib>:"WPI_AnalogChannelOpen.vi"("Analog Channel"=FPGA_AIChannel."AI 0") -> ("AIDeviceRef"=w169:T47)  [unwired: 9 in, 1 out]
  n97 = call "624ClearTalonSettings.vi"("CAN Talon SRX Ref Out"=w56) -> ("CAN Talon SRX Ref Out 2"=w57:T14)  [unwired: 10 in]
  n98 = call "624ClearTalonSettings.vi"("CAN Talon SRX Ref Out"=w58) -> ("CAN Talon SRX Ref Out 2"=w59:T14)  [unwired: 10 in]
  n99 = call <vilib>:"WPI_PotentiometerOpen.vi"("Analog Channel"=FPGA_AIChannel."AI 1") -> ("error out"=w99:errorcluster, "PotDevRef"=w98:T48)  [unwired: 9 in]
  n100 = call "624ClearTalonSettings.vi"("CAN Talon SRX Ref Out"=w60) -> ("CAN Talon SRX Ref Out 2"=w61:T14)  [unwired: 10 in]
  n101 = call <vilib>:"WPI_PotentiometerOpen.vi"("Analog Channel"=FPGA_AIChannel."AI 2") -> ("error out"=w103:errorcluster, "PotDevRef"=w102:T48)  [unwired: 9 in]
  n102 = call <vilib>:"WPI_PotentiometerOpen.vi"("Analog Channel"=FPGA_AIChannel."AI 3") -> ("error out"=w1:errorcluster, "PotDevRef"=w2:T48)  [unwired: 9 in]
  n103 = call "624ClearTalonSettings.vi"("CAN Talon SRX Ref Out"=w62) -> ("CAN Talon SRX Ref Out 2"=w63:T14)  [unwired: 10 in]
  n104 = call <vilib>:"WPI_AnalogChannelSetAveraging.vi"("OversampleBits"=u8 0, "AverageBits"=u8 5, "AIDeviceRef"=w169) -> ("AIDeviceRef"=w170:T47)  [unwired: 7 in, 1 out]
  n105 = call <vilib>:"WPI_PotentiometerRefNum Registry Set.vi"("error in (no error)"=w99, "refnum name"="Left Roller Pot", "PotDevRef"=w98) -> ()  [unwired: 7 in, 2 out]
  n106 = call <vilib>:"WPI_MotorControlRefNum Registry Set.vi"("refnum name"="Left Roller Motor", "MotorControlDevRef"=w55) -> ()  [unwired: 8 in, 2 out]
  n107 = call <vilib>:"WPI_PotentiometerRefNum Registry Set.vi"("error in (no error)"=w103, "refnum name"="Right Roller Pot", "PotDevRef"=w102) -> ()  [unwired: 7 in, 2 out]
  n108 = call <vilib>:"WPI_PotentiometerRefNum Registry Set.vi"("error in (no error)"=w1, "refnum name"="Finger Pot", "PotDevRef"=w2) -> ()  [unwired: 7 in, 2 out]
  n109 = call <vilib>:"WPI_MotorControlRefNum Registry Set.vi"("refnum name"="Right Roller Motor", "MotorControlDevRef"=w57) -> ()  [unwired: 8 in, 2 out]
  n110 = call <vilib>:"WPI_CANTalonSRX_ConfigBrakeCoast.vi"("Brake / Coast Mode"=WPI_CANTalonSRX_BrakeOverride."Override to Brake", "CAN Talon SRX Ref"=w59) -> ("CAN Talon SRX Ref"=w82:T14)  [unwired: 8 in, 1 out]
  n111 = call <vilib>:"WPI_CANTalonSRX_ConfigBrakeCoast.vi"("Brake / Coast Mode"=WPI_CANTalonSRX_BrakeOverride."Override to Brake", "CAN Talon SRX Ref"=w61) -> ("CAN Talon SRX Ref"=w85:T14)  [unwired: 8 in, 1 out]
  n112 = call <vilib>:"WPI_AnalogChannelRefNum Registry Set.vi"("refnum name"="Pressure Sensor", "AIDeviceRef"=w170) -> ()  [unwired: 8 in, 2 out]
  n113 = call <vilib>:"WPI_JoystickOpen.vi"("JoystickDevice"=WPI_JoystickDeviceEnum."USB 0") -> ("JoystickDevRef"=w178:T49)  [unwired: 10 in]
  n114 = call <vilib>:"WPI_CANTalonSRX_ConfigBrakeCoast.vi"("Brake / Coast Mode"=w64, "CAN Talon SRX Ref"=w50) -> ("CAN Talon SRX Ref"=w46:T14)  [unwired: 8 in, 1 out]
  n115 = call <vilib>:"WPI_MotorControlRefNum Registry Set.vi"("refnum name"="Center Wheel", "MotorControlDevRef"=w63) -> ()  [unwired: 8 in, 2 out]
  n116 = call <vilib>:"WPI_CANTalonSRX_ConfigBrakeCoast.vi"("Brake / Coast Mode"=w64, "CAN Talon SRX Ref"=w49) -> ("CAN Talon SRX Ref"=w68:T14)  [unwired: 8 in, 1 out]
  n117 = disable-structure shown="Enabled" {
    disable-tunnel: w85 -> [w228 w231]
    disable-tunnel: w82 -> [w227 w234]
    frame Disabled {
      n118 = call-poly <vilib>:"WPI_RobotDriveOpen2Motor.vi"("Right Motor Dev Ref"=w228, "Left Motor Dev Ref"=w227) -> ("RobotDriveDevRef"=w229:T50)  [unwired: 8 in, 1 out]
      n119 = call <vilib>:"WPI_RobotDriveRefNum Registry Set.vi"("refnum name"="Robot Wheels", "RobotDriveDevRef"=w229) -> ()  [unwired: 8 in, 2 out]
    }
    frame Enabled {
      n120 = call <vilib>:"WPI_MotorControlRefNum Registry Set.vi"("refnum name"="Drivetrain Right", "MotorControlDevRef"=w234) -> ()  [unwired: 8 in, 2 out]
      n121 = call <vilib>:"WPI_MotorControlRefNum Registry Set.vi"("refnum name"="Drivetrain Left", "MotorControlDevRef"=w231) -> ()  [unwired: 8 in, 2 out]
    }
  }
  n122 = call <vilib>:"WPI_AnalogChannelOpen.vi"("Analog Channel"=FPGA_AIChannel."AI 3") -> ("error out"=w5:errorcluster, "AIDeviceRef"=w7:T47)  [unwired: 9 in]
  n123 = call <vilib>:"WPI_JoystickOpen.vi"("JoystickDevice"=WPI_JoystickDeviceEnum."USB 1") -> ("JoystickDevRef"=w151:T49)  [unwired: 10 in]
  n124 = call <vilib>:"WPI_CANTalonSRX_ConfigLimitSwitches.vi"("CAN Talon SRX Ref"=w68, "Forward Limit Switch Normally Open"=w66, "Reverse Limit Switch Normally Open"=w66, "error in (no error)"=errorcluster {"status"=FALSE, "code"=0, "source"=""}) -> ("CAN Talon SRX Ref"=w70:T14, "error out"=w69:errorcluster)  [unwired: 10 in]
  n125 = call <vilib>:"WPI_JoystickRefNum Registry Set.vi"("refnum name"="Manipulator", "JoystickDevRef"=w151) -> ()  [unwired: 8 in, 2 out]
  n126 = call <vilib>:"WPI_JoystickRefNum Registry Set.vi"("refnum name"="Driver", "JoystickDevRef"=w178) -> ()  [unwired: 8 in, 2 out]
  n127 = call <vilib>:"WPI_AnalogChannelSetSampleRate.vi"("Samples Per Second (per channel)"=1000.0) -> ()  [unwired: 10 in, 1 out]
  n128 = call <vilib>:"WPI_AnalogChannelRefNum Registry Set.vi"("error in (no error)"=w5, "refnum name"="Finger Pot", "AIDeviceRef"=w7) -> ()  [unwired: 7 in, 2 out]
  n129 = call <vilib>:"WPI_MotorControlRefNum Registry Set.vi"("refnum name"="Elevator Slave", "MotorControlDevRef"=w46) -> ()  [unwired: 8 in, 2 out]
  n130 = call <vilib>:"WPI_MotorControlRefNum Registry Set.vi"("error in (no error)"=w69, "refnum name"="Elevator", "MotorControlDevRef"=w70) -> ()  [unwired: 7 in, 2 out]
  n131 = disable-structure shown="Disabled" {
    frame Disabled {
      n132 = call-poly <vilib>:"WPI_UltrasonicOpen.vi"("Echo DIO Channel"=FPGA_DIOChannel."DIO 7", "Ping DIO Channel"=FPGA_DIOChannel."DIO 6") -> ("error out"=w239:errorcluster, "SonarSRF04DevRef"=w238:T51)  [unwired: 8 in]
      n133 = call-poly <vilib>:"WPI_UltrasonicOpen.vi"("Echo DIO Channel"=FPGA_DIOChannel."DIO 9", "Ping DIO Channel"=FPGA_DIOChannel."DIO 8") -> ("error out"=w244:errorcluster, "SonarSRF04DevRef"=w243:T51)  [unwired: 8 in]
      n134 = call-poly <vilib>:"WPI_UltrasonicRefNum Registry Set.vi"("error in (no error)"=w239, "refnum name"="Left Ping Sensor", "SonarSRF04DevRef"=w238) -> ()  [unwired: 7 in, 2 out]
      n135 = call-poly <vilib>:"WPI_UltrasonicRefNum Registry Set.vi"("error in (no error)"=w244, "refnum name"="Right Ping Sensor", "SonarSRF04DevRef"=w243) -> ()  [unwired: 7 in, 2 out]
    }
    frame Enabled {
    }
  }
  n136 = call <vilib>:"WPI_AnalogOutputOpen.vi"("AO Channel"=WPI_AnalogOutputChannel."AO MXP 0") -> ("error out"=w23:errorcluster, "AODeviceRef"=w24:T52)  [unwired: 9 in]
  n137 = call <vilib>:"WPI_DigitalOutputOpen.vi"("DIO Channel"=FPGA_DIOChannel."DIO 7") -> ("error out"=w12:errorcluster, "DigitalOutputDevRef"=w11:T53)  [unwired: 9 in]
  n138 = call <vilib>:"WPI_AnalogOutputOpen.vi"("AO Channel"=WPI_AnalogOutputChannel."AO MXP 1") -> ("error out"=w21:errorcluster, "AODeviceRef"=w18:T52)  [unwired: 9 in]
  n139 = call <vilib>:"WPI_DigitalOutputOpen.vi"("DIO Channel"=FPGA_DIOChannel."DIO 8") -> ("error out"=w13:errorcluster, "DigitalOutputDevRef"=w14:T53)  [unwired: 9 in]
  n140 = call <vilib>:"WPI_DigitalOutputOpen.vi"("DIO Channel"=FPGA_DIOChannel."DIO 9") -> ("error out"=w28:errorcluster, "DigitalOutputDevRef"=w27:T53)  [unwired: 9 in]
  n141 = call <vilib>:"WPI_DigitalOutputRefNum Registry Set.vi"("error in (no error)"=w12, "refnum name"="State 3", "DigitalOutputDevRef"=w11) -> ()  [unwired: 7 in, 2 out]
  n142 = call <vilib>:"WPI_AnalogOutputRefNum Registry Set.vi"("error in (no error)"=w23, "refnum name"="FingerHeight", "AODeviceRef"=w24) -> ()  [unwired: 7 in, 2 out]
  n143 = call <vilib>:"WPI_DigitalOutputRefNum Registry Set.vi"("error in (no error)"=w13, "refnum name"="State 2", "DigitalOutputDevRef"=w14) -> ()  [unwired: 7 in, 2 out]
  n144 = call <vilib>:"WPI_DigitalOutputRefNum Registry Set.vi"("error in (no error)"=w28, "refnum name"="State 1", "DigitalOutputDevRef"=w27) -> ()  [unwired: 7 in, 2 out]
  n145 = call <vilib>:"WPI_AnalogOutputRefNum Registry Set.vi"("error in (no error)"=w21, "refnum name"="Multiplexer", "AODeviceRef"=w18) -> ()  [unwired: 7 in, 2 out]
  n146 = call-poly <vilib>:"WPI_UltrasonicOpen.vi"("Echo DIO Channel"=FPGA_DIOChannel."DIO 5", "Ping DIO Channel"=FPGA_DIOChannel."DIO 4") -> ("error out"=w74:errorcluster, "SonarSRF04DevRef"=w75:T51)  [unwired: 8 in]
  n147 = call-poly <vilib>:"WPI_UltrasonicRefNum Registry Set.vi"("error in (no error)"=w74, "refnum name"="Center Ping Sensor", "SonarSRF04DevRef"=w75) -> ()  [unwired: 7 in, 2 out]
